vi "Read Selection.vi"(8 "error in (no error)":errorcluster, 11 "ListSelection in":refnum<class "ListSelection.lvclass">) -> (0 "error out":errorcluster, 2 "Selection":i32[](array[numeric]), 3 "ListSelection out":refnum<class "ListSelection.lvclass">)   [LabVIEW 2012, in "ListSelection.lvlib" / "ListSelection.lvclass"]
uses:
  ListSelection.lvclass
  ListSelection.lvclass/ListSelection.ctl
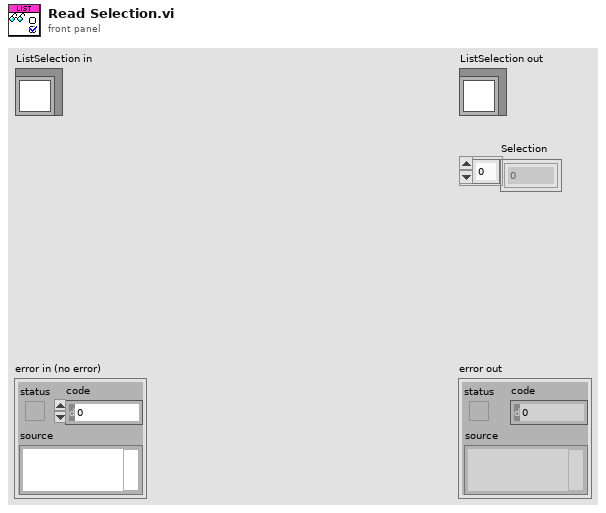
[diagram p1: front panel]
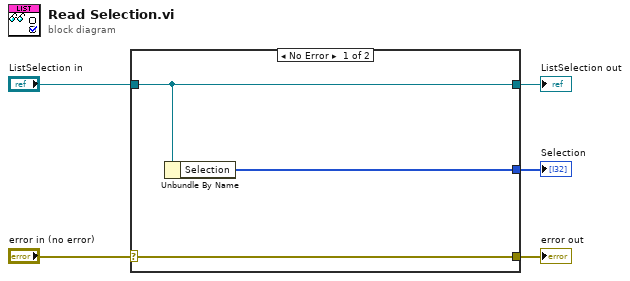
[diagram p0: block diagram]
diagram:
  n1 = case shown="No Error" "error in (no error)" {
    selector: "error in (no error)" -> [w8 w9]
    tunnel: [w8 w9] -> w4
    tunnel: [w7 w10] -> w2
    tunnel: "ListSelection in" -> [w7 w10]
    tunnel: [w6 _] -> w1
    frame No Error {
      n2 = Unbundle By Name(w7) -> ("Selection"=w6:i32[])
    }
    frame Error {
    }
  }
  "error out" <- w4
  "ListSelection out" <- w2
  "Selection" <- w1
